vi "Trigger Detector.vi"(0 "phasors":csg[](array[numeric]), 1 "triggers definition":T2={"magnitudes and phases"=[], "frequency high limit [Hz]"=70.0, "frequency low limit [Hz]"=40.0, "df/dt limit [Hz/s]"=323.67}, 2 "reset? (F)":bool, 5 "frequency":sgl, 7 "df/dt":sgl, 11 "error in (no error)":errorcluster) -> (4 "triggers":T1, 6 "trigger reason":u8=8 format="%04b", 15 "error out":errorcluster)   [LabVIEW 2013, in "NI_EP_PMU.lvlib"]
doc: "Detects triggers and returns the bitmapped flags of trigger reason in the STAT field of the data frame as defined in IEEE Std C37.118.2-2011."
uses:
  <vilib>/addons/Electrical Power/PMU/NI_EP_PMU.lvlib
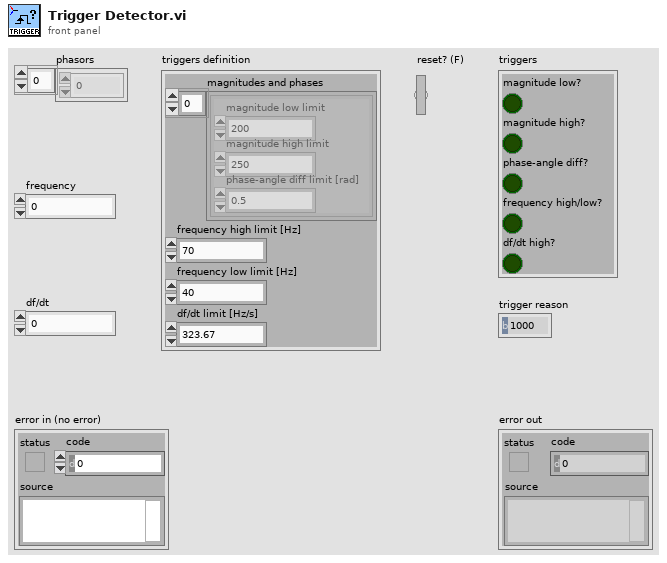
[diagram p1: front panel]
types:
  T1 = cluster{"magnitude low?":bool, "magnitude high?":bool, "phase-angle diff?":bool, "frequency high/low?":bool, "df/dt high?":bool}
  T2 = cluster{"magnitudes and phases":cluster{"magnitude low limit":sgl, "magnitude high limit":sgl, "phase-angle diff limit [rad]":sgl}[], "frequency high limit [Hz]":sgl, "frequency low limit [Hz]":sgl, "df/dt limit [Hz/s]":sgl}
  T3 = cluster{"magnitude low":bool, "magnitude high":bool, "phase-angle diff":bool, "frequency high/low":bool, "df/dt high":bool}
  T4 = cluster{"magnitude and phase":cluster{"mag. lower limit":sgl, "mag.upper limit":sgl, "phase diff limit (radian)":sgl}[], "freq. upper limit (Hz)":sgl, "freq. lower limit (Hz)":sgl, "rate of change limit (Hz/s)":sgl}
  T5 = cluster{"mag. lower limit":sgl, "mag.upper limit":sgl, "phase diff limit (radian)":sgl}[]
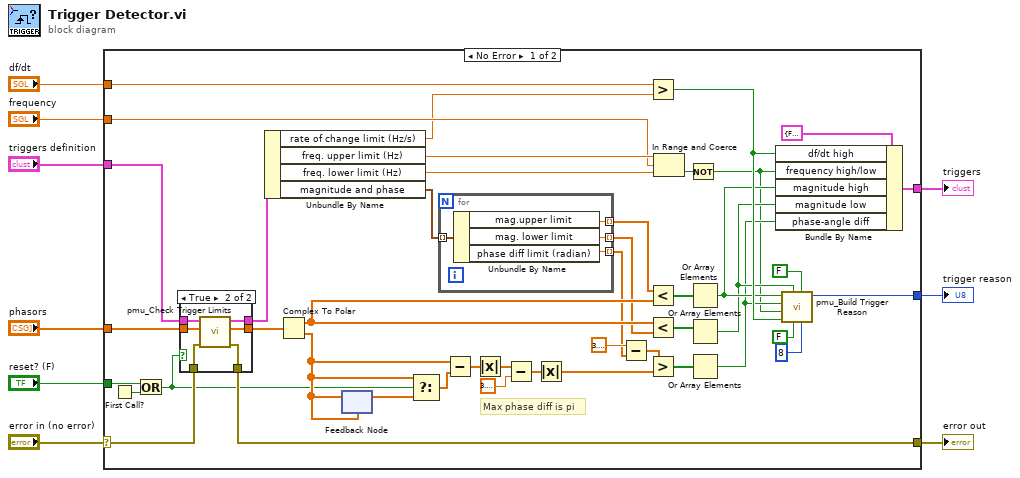
[diagram p0: block diagram]
diagram:
  n1 = case shown="No Error" "error in (no error)" {
    selector: "error in (no error)" -> [w14 w67]
    tunnel: "phasors" -> [w12 _]
    tunnel: "triggers definition" -> [w16 _]
    tunnel: "frequency" -> [w50 _]
    tunnel: "df/dt" -> [w47 _]
    tunnel: [w13 w67] -> w4
    tunnel: [w38 _] -> w3
    tunnel: [w29 _] -> w2
    tunnel: "reset? (F)" -> [w24 _]
    frame No Error {
      # "Max phase diff is pi"
      n2 = First Call?() -> (First Call?: T/F=w25:bool)
      n3 = Or(x=w24, y=w25) -> (x .or. y?=w10:bool)
      n4 = case shown="True" w10 {
        tunnel: w16 -> [w56 w62]
        tunnel: [w56 w61] -> w15
        tunnel: w14 -> [w54 w60]
        tunnel: [w54 w59] -> w13
        tunnel: w12 -> [w55 w58]
        tunnel: [w55 w57] -> w11
        frame False {
        }
        frame True {
          n5 = call <vilib>:"pmu_Check Trigger Limits.vi"("error in (no error)"=w60, "phasors in"=w58, "trigger limits in"=w62) -> ("error out"=w59:errorcluster, "phasors out"=w57:csg[], "trigger limits out"=w61:T4)  [unwired: 6 in]
        }
      }
      n6 = Unbundle By Name(w15) -> ("rate of change limit (Hz/s)"=w46:sgl, "freq. upper limit (Hz)"=w52:sgl, "freq. lower limit (Hz)"=w51:sgl, "magnitude and phase"=w48:T5)
      n7 = Complex To Polar(r * e^(i*theta)=w11) -> (r=w44:sgl[], theta=w28:sgl[])
      n8 = feedback-in #1(w28) -> ()
      n9 = feedback #1(w28) -> (w27:sgl[])
      n10 = Select(t=w28, s=w10, f=w27) -> (s? t:f=w26:sgl[])
      n11 = for {
        tunnel: w48 -> [w66] mode=indexing
        tunnel: [w65] -> w45 mode=indexing
        tunnel: [w64] -> w43 mode=indexing
        tunnel: [w63] -> w18 mode=indexing
        n12 = Unbundle By Name(w66) -> ("mag.upper limit"=w65:sgl, "mag. lower limit"=w64:sgl, "phase diff limit (radian)"=w63:sgl)
      }
      n13 = Subtract(x=w28, y=w26) -> (x-y=w53:sgl[])
      n14 = Absolute Value(x=w53) -> (abs(x)=w23:sgl[])
      n15 = Subtract(x=w23, y=sgl 3.1415927) -> (x-y=w21:sgl[])
      n16 = Absolute Value(x=w21) -> (abs(x)=w20:sgl[])
      n17 = Subtract(x=sgl 3.1415927, y=w18) -> (x-y=w17:sgl[])
      n18 = Greater?(x=w47, y=w46) -> (0:w37:bool)
      n19 = Less?(x=w45, y=w44) -> (x < y?=w42:bool[])
      n20 = Less?(x=w44, y=w43) -> (x < y?=w41:bool[])
      n21 = Greater?(x=w17, y=w20) -> (0:w40:bool[])
      n22 = In Range and Coerce(upper limit=w52, x=w50, lower limit=w51) -> (In Range?=w49:bool)  [unwired: 1 out]
      n23 = Not(x=w49) -> (.not. x?=w33:bool)
      n24 = Or Array Elements(Boolean array=w42) -> (logical OR=w36:bool)
      n25 = Or Array Elements(Boolean array=w41) -> (logical OR=w35:bool)
      n26 = Or Array Elements(Boolean array=w40) -> (logical OR=w34:bool)
      n27 = Bundle By Name(cluster=T3 {"magnitude low"=FALSE, "magnitude high"=FALSE, "phase-angle diff"=FALSE, "frequency high/low"=FALSE, "df/dt high"=FALSE} ("trigger detected"), "df/dt high"=w37, "frequency high/low"=w33, "magnitude high"=w36, "magnitude low"=w35, "phase-angle diff"=w34) -> (w38:T3)
      n28 = call <vilib>:"pmu_Build Trigger Reason.vi"("user defined trigger reason"=u8 8, "manual"=FALSE, "digital"=FALSE, "magnitude low"=w35, "df/dt high"=w37, "frequency high/low"=w33, "phase-angle diff"=w34, "magnitude high"=w36) -> ("trigger reason"=w29:u8)  [unwired: 3 in]
    }
    frame Error {
    }
  }
  "error out" <- w4
  "triggers" <- w3
  "trigger reason" <- w2
